vi "Register Events to Source.vi"(8 "error in (no error)":errorcluster, 11 "Example Sink in":refnum<class "Example Sink.lvclass">) -> (0 "error out":errorcluster, 3 "Example Sink out":refnum<class "Example Sink.lvclass">)   [LabVIEW 2016, in "Example Sink.lvlib" / "Example Sink.lvclass"]
doc: "This dinamic dispatch methods has to be overriddent by the child sink classes to register events to the source"
uses:
  Example Sink.lvclass
  C:/Projects/Shared Libraries/Event Actors/Event Sink/Event Sink.lvclass
  Alternative Example Sink/Example Sink Messages/Update Array Msg/Update Array Msg.lvclass
  C:/Projects/Shared Libraries/Event Actors/Event Source Messages/Event Generated Msg/Event Generated Msg.lvclass
  Example Source/Example Events/Double Array Event.lvclass
  C:/Projects/Shared Libraries/Event Actors/Event/Event.lvclass
  Alternative Example Sink/Example Sink Messages/Update Time Msg/Update Time Msg.lvclass
  Example Source/Example Events/Timestamp Event.lvclass
  Alternative Example Sink/Example Sink Messages/Update Boolean Msg/Update Boolean Msg.lvclass
  Example Source/Example Events/Boolean Event.lvclass
  Event/Event.lvclass/Event.ctl
  Event Sink/Event Sink.lvclass/Event Sink.ctl
  Event Sink/properties/Read Event Source Enqueuer.vi
  Event Sink/properties/Read Name.vi
  <vilib>/ActorFramework/Message Enqueuer/Message Enqueuer.lvclass
  Event/Event.lvclass
  Event Source Messages/Register by Name Msg/Register by Name Msg.lvclass
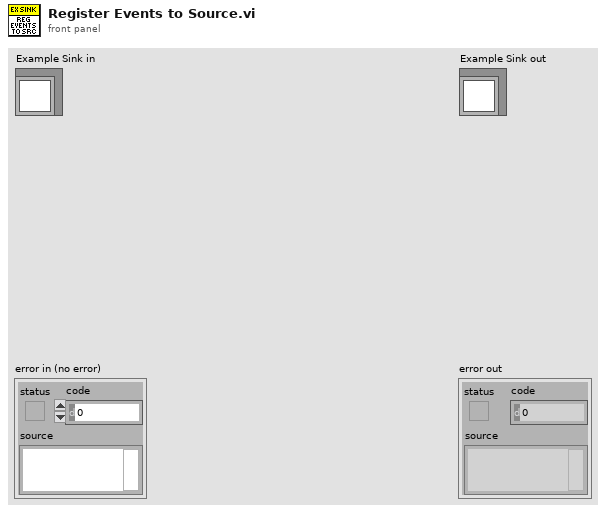
[diagram p1: front panel]
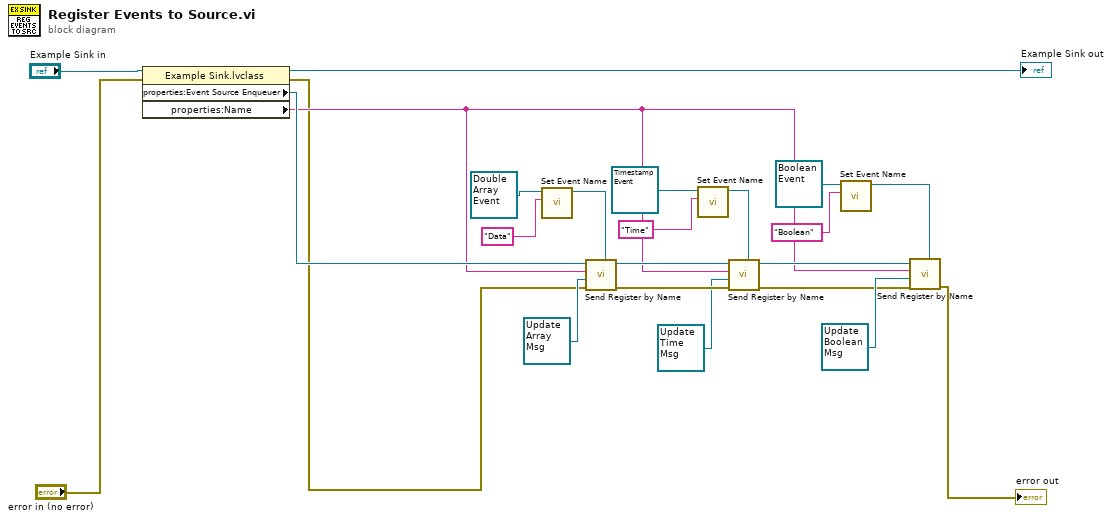
[diagram p0: block diagram]
diagram:
  n1 = property class="Example Sink.lvclass"(reference="Example Sink in", error in="error in (no error)") -> (reference out=→"Example Sink out":refnum<class "Example Sink.lvclass">, error out=w2:errorcluster, "properties:Event Source Enqueuer"=w5:refnum<class "Message Enqueuer.lvclass">, "properties:Name"=w4:string)
  n2 = call "Set Event Name.vi"("Name (Generic)"="Data", "Event In"=refnum<class "Double Array Event.lvclass"> refnum ("Double Array Event.lvclass")) -> ("Event Out"=w16:refnum<class "Double Array Event.lvclass">)  [unwired: 9 in]
  n3 = call "Send Register by Name.vi"("Event"=w16, "error in (no error)"=w2, "Event Fire Handler"=refnum<class "Update Array Msg.lvclass"> refnum ("Update Array Msg.lvclass"), "Sink Name"=w4, "Message Enqueuer in"=w5) -> ("error out"=w10:errorcluster, "Message Enqueuer out"=w12:refnum<class "Message Enqueuer.lvclass">)  [unwired: 5 in]
  n4 = call "Set Event Name.vi"("Name (Generic)"="Time", "Event In"=refnum<class "Timestamp Event.lvclass"> refnum ("Timestamp Event.lvclass")) -> ("Event Out"=w7:refnum<class "Timestamp Event.lvclass">)  [unwired: 9 in]
  n5 = call "Send Register by Name.vi"("Event"=w7, "error in (no error)"=w10, "Event Fire Handler"=refnum<class "Update Time Msg.lvclass"> refnum ("Update Time Msg.lvclass"), "Sink Name"=w4, "Message Enqueuer in"=w12) -> ("error out"=w9:errorcluster, "Message Enqueuer out"=w11:refnum<class "Message Enqueuer.lvclass">)  [unwired: 5 in]
  n6 = call "Set Event Name.vi"("Name (Generic)"="Boolean", "Event In"=refnum<class "Boolean Event.lvclass"> refnum ("Example Source.lvlib:Boolean Event.lvclass")) -> ("Event Out"=w14:refnum<class "Boolean Event.lvclass">)  [unwired: 9 in]
  n7 = call "Send Register by Name.vi"("Event"=w14, "error in (no error)"=w9, "Event Fire Handler"=refnum<class "Update Boolean Msg.lvclass"> refnum ("Update Time Msg.lvclass"), "Sink Name"=w4, "Message Enqueuer in"=w11) -> ("error out"=→"error out":errorcluster)  [unwired: 5 in, 1 out]
